vi "mtoloader.vi"(11 "m":dbl) -> (3 "loader":dbl)   [LabVIEW 2019]
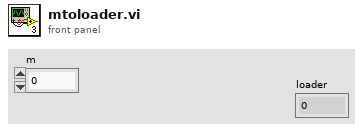
[diagram p1: front panel]
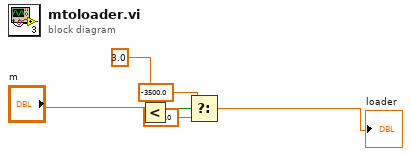
[diagram p0: block diagram]
diagram:
  n1 = Less?(x="m", y=3.0) -> (x < y?=w6:bool)
  n2 = Select(t=-3500.0, s=w6, f=-2500.0) -> (s? t:f=→"loader":dbl)
